vi "SparkFun Motor Driver.vi"() -> ()   [LabVIEW 2019]
uses:
  <userlib>/MicroPython/VIs/uPythonX/uPythonX.xctl
panel:
  in  "Tab Control":T1(tab)=enum."WeDo"
  in  "Motors":T2(xcontrol)={"VISA Refnum in"="ASRL23::INSTR", "Python Code"="# In 1    In2    PWM   Out1    Out2    Mode\n#   H       H       H/L       L          L        short break\n#   L        H         H        L          H        CCW\n#   L        H         L        L          H        short break\n#   H        L         H       H          L        CW\n#   H        L         L        L          H       short break\n#   L         L         L        L          L        Stop\n\n# STBY must be high\n\nfrom pyb import Pin, Timer\n\nA_PWM = Pin('W29') # W29 has TIM2, CH2\nAIn2 = Pin('W22', Pin.OUT)\nAIn1 = Pin('W16',Pin.OUT)\nStdby = Pin('W24',Pin.OUT)\n\nBIn1 = Pin('Y12', Pin.OUT)\nBIn2 = Pin('W32',Pin.OUT)\nB_PWM = Pin('Y11') #  TIM8, CH2\n\ntimA = Timer(2, freq=1000)\ntimB = Timer(8, freq=1000)\n\nSpeedA = -50\nSpeedB = 50\n\nStdby.value(0)  #turn motors off until reset\n\nif (SpeedA < 0):\n     AIn1.value(255)\n     AIn2.value(0)\n     SpeedA = - SpeedA\nelse:\n     AIn1.value(0)\n     AIn2.value(255)\n\nif (SpeedB < 0):\n     BIn1.value(255)\n     BIn2.value(0)\n     SpeedB = - SpeedB\nelse:\n     BIn1.value(0)\n     BIn2.value(255)\n\nchA = timA.channel(2, Timer.PWM, pin= A_PWM)\nchA.pulse_width_percent(SpeedA)\nchB = timB.channel(2, Timer.PWM, pin= B_PWM)\nchB.pulse_width_percent(SpeedB)\n\nStdby.value(255)  #everything is ready - reset motors\n"}
  in  "Tacho":T2(xcontrol)={"VISA Refnum in"="ASRL23::INSTR", "Python Code"="# Old |      New Value\n#        |    0    1   2   3\n#   0   |    0   -1  1   X\n#   1   |    1    0   X  -1\n#   2   |   -1   X   0   1\n#   3   |    X    1  -1  0\n\n\n# From https://cdn.sparkfun.com/datasheets/Robotics/How%20to%20use%20a%20quadrature%20encoder.pdf\n\nfrom pyb import Pin\nimport array\nimport utime\n\nM1_New = 0\nM1_EncA = Pin('Y1', Pin.IN, pull = Pin.PULL_UP)\nM1_EncB = Pin('Y2', Pin.IN, pull = Pin.PULL_UP)\n\nM1_Matrix = array.array('l',[0,-1,1,2,1,0,2,-1,-1,2,0,1,2,1,-1,0])\n\n#To read the array my index is: Old * 4 + New So my code reads like this:\nwhile True:\n     M1_Old = M1_New\n     M1_New = M1_EncA.value()  * 2 + M1_EncB.value()\n     Out = M1_Matrix [M1_Old * 4 + M1_New]\n     print('Old: %2d   New: %2d    Out %2d' % (M1_Old, M1_New, Out))\n     utime.sleep(0.01)\n"}
  in  "Tacho 2":T2(xcontrol)={"VISA Refnum in"="ASRL23::INSTR", "Python Code"="# From https://github.com/peterhinch/micropython-samples/blob/master/encoders/encoder.py\n\nfrom pyb import Pin\nimport utime\n\nclass Encoder(object):\n    def __init__(self, pin_x, pin_y, reverse, scale):\n        self.reverse = reverse\n        self.scale = scale\n        self.forward = True\n        self.pin_x = pin_x\n        self.pin_y = pin_y\n        self._pos = 0\n        self.x_interrupt = pyb.ExtInt(pin_x, pyb.ExtInt.IRQ_RISING_FALLING, pyb.Pin.PULL_NONE, self.x_callback)\n        self.y_interrupt = pyb.ExtInt(pin_y, pyb.ExtInt.IRQ_RISING_FALLING, pyb.Pin.PULL_NONE, self.y_callback)\n\n    def x_callback(self, line):\n        self.forward = self.pin_x.value() ^ self.pin_y.value() ^ self.reverse\n        self._pos += 1 if self.forward else -1\n\n    def y_callback(self, line):\n        self.forward = self.pin_x.value() ^ self.pin_y.value() ^ self.reverse ^ 1\n        self._pos += 1 if self.forward else -1\n\n    @property\n    def position(self):\n        return self._pos*self.scale\n\n    def reset(self):\n        self._pos = 0\n\npin1 = Pin('Y4', Pin.IN)\npin2 = Pin('Y3', Pin.IN)\n\ne=Encoder(pin1,pin2,False,0.5)\ne.reset()\nwhile True:\n     e.position\n     utime.sleep(1)"}
  in  "PyBoard":T2(xcontrol)={"VISA Refnum in"="ASRL23::INSTR", "Python Code"="import time,pyb\n\nuart = pyb. UART(3,9600, bits=8, parity=None, stop=1)\n\nwhile(True):\n    time.sleep_ms(100)\n    size = uart.any()\n    if (size > 0):\n        string = uart.read(size)\n        data = int(string[-1])\n        print('Data: %3d' % (data))\n\n\n"}
  in  "Camera":T2(xcontrol)={"VISA Refnum in"="ASRL12::INSTR", "Python Code"="# Show intensity mean\n\nimport sensor, image, time\nimport pyb\n\nclock = time.clock()\nsensor.reset()\nsensor.set_pixformat(sensor.RGB565)\nsensor.set_framesize(sensor.QVGA)\nsensor.skip_frames(time = 2000)\nsensor.set_auto_gain(True)\nsensor.set_auto_whitebal(True) \n\n\nuart = pyb.UART(3,9600, bits=8, parity=None, stop=1)\n\nprint('Starting...')\nwhile(True):\n    clock.tick()\n    img = sensor.snapshot()\n    data = img.statistics()[0]\n    end = uart.write(chr(data))\n"}
  in  "WeDo":T2(xcontrol)={"VISA Refnum in"="ASRL12::INSTR", "Python Code"="import machine, utime, gc\nimport sensor, image\n\ndef send_value(data):\n     value = (data & 0xFF)\n     payload = bytes([0xC0, value, 0xFF ^ 0xC0 ^ value])\n     uart.write(payload)\n\n# Show intensity mean\ndef camera():\n     sensor.reset()\n     sensor.set_pixformat(sensor.RGB565)\n     sensor.set_framesize(sensor.QVGA)\n     sensor.skip_frames(time = 2000)\n     sensor.set_auto_gain(True)\n     sensor.set_auto_whitebal(True) \n     \ncamera()\n\ntx = machine.Pin('P4', machine.Pin.OUT)\nrx = machine.Pin('P5', machine.Pin.IN)\ntx.value(0)\nutime.sleep_ms(500)\ntx.value(1)\n\nuart = machine.UART(3)\nuart.init(baudrate=2400, bits=8, parity=None, stop=1)\n\nuart.write(b'\\x00')\nuart.write(b'\\x40\\x23\\x9C')\nuart.write(b'\\x49\\x02\\x01\\xB5')\nuart.write(b'\\x52\\x00\\xC2\\x01\\x00\\x6E')\nuart.write(b'\\x5F\\x00\\x00\\x00\\x02\\x00\\x00\\x00\\x02\\xA0')\nuart.write(b'\\x9A\\x00\\x4C\\x50\\x46\\x32\\x2D\\x43\\x41\\x4C\\x6E')\nuart.write(b'\\x9A\\x01\\x00\\x00\\x00\\x00\\x00\\xC0\\x7F\\x44\\x9F')\nuart.write(b'\\x9A\\x02\\x00\\x00\\x00\\x00\\x00\\x00\\xC8\\x42\\xED')\nuart.write(b'\\x9A\\x03\\x00\\x00\\x00\\x00\\x00\\xC0\\x7F\\x44\\x9D')\nuart.write(b'\\x92\\x04\\x52\\x41\\x57\\x00\\x2D')\nuart.write(b'\\x8A\\x05\\x10\\x00\\x60')\nuart.write(b'\\x92\\x80\\x03\\x01\\x03\\x00\\xEC')\nutime.sleep_ms(5)\nprint(uart.read(uart.any()))\nuart.write(b'\\xA1\\x00\\x4C\\x50\\x46\\x32\\x2D\\x43\\x4F\\x55\\x4E\\x54\\x00\\x00\\x00\\x00\\x00\\x00\\x58')\nuart.write(b'\\x99\\x01\\x00\\x00\\x00\\x00\\x00\\x00\\xC8\\x42\\xED')\nuart.write(b'\\x99\\x02\\x00\\x00\\x00\\x00\\x00\\x00\\xC8\\x42\\xEE')\nuart.write(b'\\x99\\x03\\x00\\x00\\x00\\x00\\x00\\x00\\xC8\\x42\\xEF')\nuart.write(b'\\x91\\x04\\x43\\x4E\\x54\\x00\\x33')\nuart.write(b'\\x89\\x05\\x10\\x00\\x63')\nuart.write(b'\\x91\\x80\\x01\\x02\\x04\\x00\\xE9')\nutime.sleep_ms(5)\nprint(uart.read(uart.any()))\nuart.write(b'\\xA0\\x00\\x4C\\x50\\x46\\x32\\x2D\\x44\\x45\\x54\\x45\\x43\\x54\\x00\\x00\\x00\\x00\\x00\\x1D')\nuart.write(b'\\x98\\x01\\x00\\x00\\x00\\x00\\x00\\x00\\x20\\x41\\x07')\nuart.write(b'\\x98\\x02\\x00\\x00\\x00\\x00\\x00\\x00\\xC8\\x42\\xEF')\nuart.write(b'\\x98\\x03\\x00\\x00\\x00\\x00\\x00\\x00\\x20\\x41\\x05')\nuart.write(b'\\x80\\x04\\x00\\x7B')\nuart.write(b'\\x88\\x05\\x10\\x00\\x62')\nuart.write(b'\\x90\\x80\\x01\\x00\\x03\\x00\\xED')\nutime.sleep_ms(5)\nprint(uart.read(uart.any()))\nuart.write(b'\\x04')\n\n# wait for ACK\nstarttime = utime.time()\ncurrenttime = starttime\n\nwhile (currenttime-starttime) < 2000:\n     utime.sleep_ms(5)\n     data = uart.read(uart.any())\n     if data.find(b'\\x04') >= 0:\n          print('Success')\n          currenttime = starttime+3000   # stop the loop\n     else:\n          currenttime = utime.time()\n\n# pull pin low\nuart.deinit()\ntx = machine.Pin('P4', machine.Pin.OUT)\ntx.value(0)\nutime.sleep_ms(10)\n\n#change baudrate\n\nuart.init(baudrate=115200, bits=8, parity=None, stop=1)\n\n# loop from -10 to 10\ni=0\n\nwhile True:\n     gc.collect()\n     img = sensor.snapshot()\n     data = img.statistics()[0]\n     send_value(data)\n     i += 1\n     if i > 10: i=-10\n     utime.sleep_ms(200)\n"}
  in  "Test 2":T2(xcontrol)={"VISA Refnum in"="ASRL23::INSTR", "Python Code"="# from https://docs.micropython.org/en/latest/reference/isr_rules.html\n\nimport pyb, micropython\nmicropython.alloc_emergency_exception_buf(100)  # this makes verbose debugging\n\n\nclass LightShow(object):\n    def __init__(self,timer, led):\n        self.led = led\n        timer.callback(self.ToggleIt)\n    def ToggleIt (self,line):\n        self.led.toggle()\n\ntimer1 = pyb.Timer(4, freq=1)\ntimer2 = pyb.Timer(2, freq=0.8)\nled1 =  pyb.LED(1)\nled2 = pyb.LED(2)\n\nred = LightShow(timer1,led1)\ngreen = LightShow(timer2,led2 )\n\n\n# you need to hit Ctrl D to stop the interrupts\n"}
  # "Motor1"
  # "Motor2"
  # "Tx"
  # "Rx"
  # "3.3V"
  # "GRND"
  # "Blue"
  # "Green"
  # "Yellow"
  # "Red"
  # "Orange"
  # "Magenta"
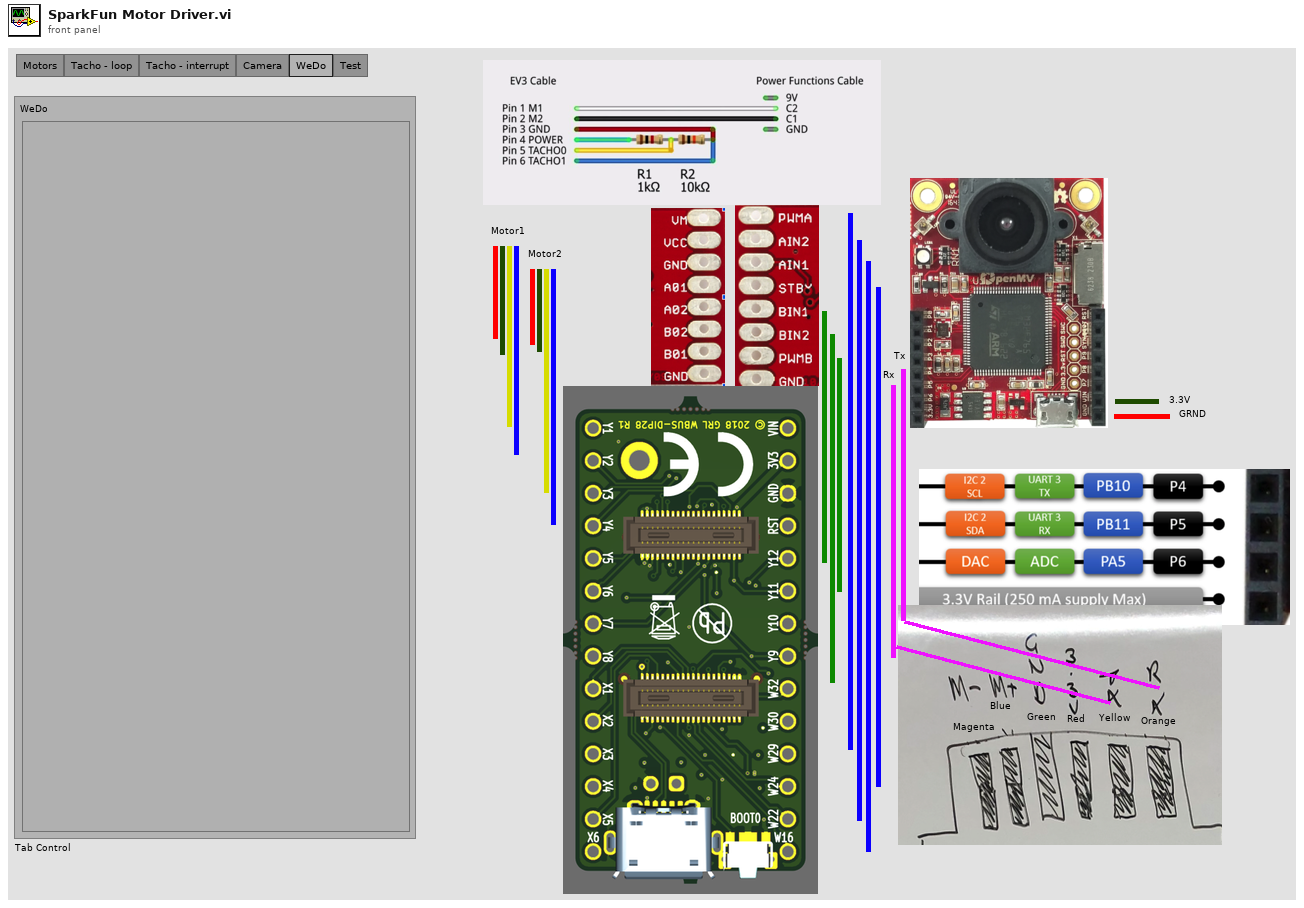
[diagram p1: front panel]
types:
  T1 = enum32{"Motors", "Tacho - loop", "Tacho - interrupt", "Camera", "WeDo", "Test"}
  T2 = cluster{"VISA Refnum in":refnum<visa-resource-name>, "Python Code":string}
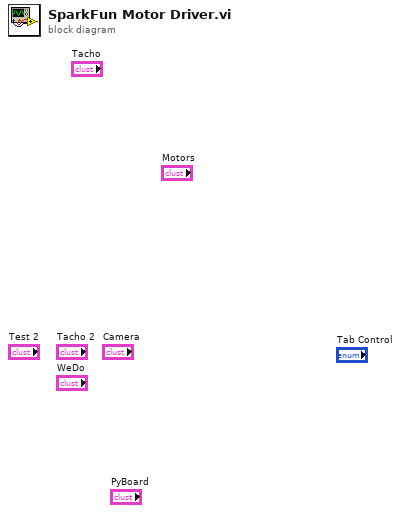
[diagram p0: block diagram]
diagram:
